vi "PNA-X control.vi"() -> ()   [LabVIEW 2020, in "VNA-Keysight PNA.lvclass"]
uses:
  VNA-Keysight PNA.lvclass
  <instrlib>/Keysight PNA Series/Keysight PNA Series.lvlib
panel:
  out "XY Graph":cluster{dbl[], dbl[]}(graph)
  in  "Sweep Points (201)":i32=201
  out "Data":dbl[](graph)
  in  "Stop Frequency (1E+10 Hz)":dbl=10000000000.0
  in  "Start Frequency (1E+6 Hz)":dbl=1000000.0
  in  "Measurement Name (MyMeas)":string="MyMeas"
  in  "Measurement Parameters (S22)":string="S22"
  in  "Channel (1)":i32=1
  in  "VISA resource name":refnum<visa-resource-name>
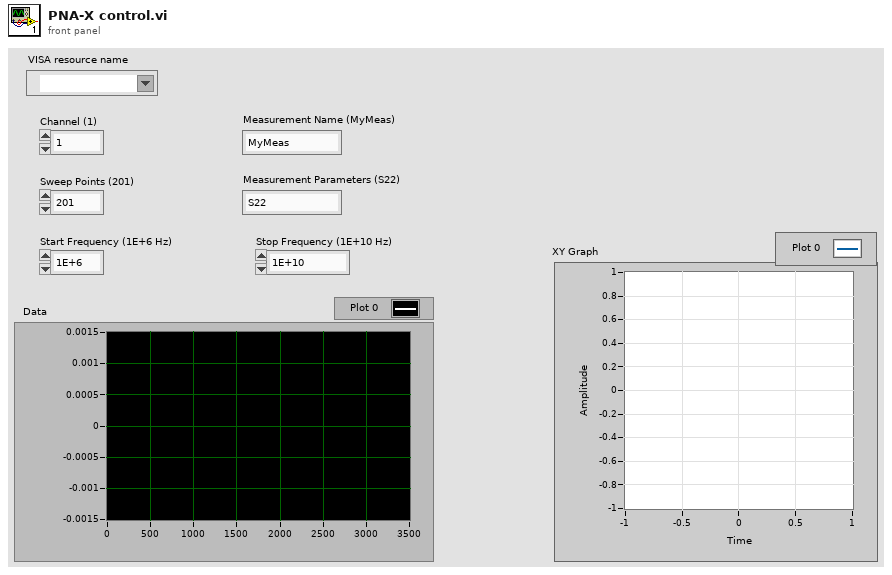
[diagram p1: front panel]
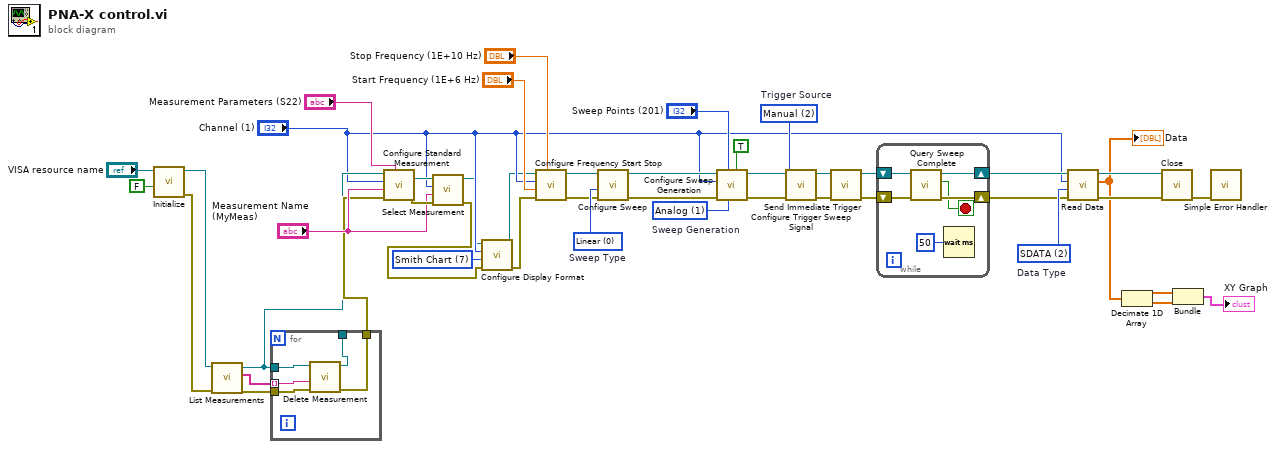
[diagram p0: block diagram]
diagram:
  w5 = 7 items=["Magnitude Linear", "Magnitude Logarithmic", "Phase", "Unwrapped phase", "Imaginary", "Real", "Polar", "Smith Chart", "Smith Admittance", "SWR", "Group Delay", "Kelvin", "Fahrenheit", "Celsius"] ("Display Format (0: Magnitude Linear)")
  w20 = 2 items=["Immediate", "External", "Manual"]  # Trigger Source
  w27 = 1 items=["Stepped", "Analog"]  # Sweep Generation
  w34 = 2 items=["FDATA", "RDATA", "SDATA", "FMEM", "SMEM", "SDIV"]  # Data Type
  w39 = 0 items=["Linear", "Logarithmic", "Power", "CW", "Segment", "Phase"]  # Sweep Type
  n1 = call <instrlib>:"Initialize.vi"("Reset (True)"=FALSE, "VISA resource name"="VISA resource name") -> ("error out"=w9:errorcluster, "VISA resource name out"=w10:refnum<visa-resource-name>)  [unwired: 8 in]
  n2 = call <instrlib>:"List Measurements.vi"("error in (no error)"=w9, "VISA resource name"=w10) -> ("error out"=w12:errorcluster, "Measurement Names"=w11:string[], "VISA resource name out"=w7:refnum<visa-resource-name>)  [unwired: 6 in, 1 out]
  n3 = for {
    tunnel: w7 -> [w50]
    tunnel: w12 -> [w49]
    tunnel: w11 -> [w48] mode=indexing
    tunnel: [w47] -> _
    tunnel: [w46] -> w8
    n4 = call <instrlib>:"Delete Measurement.vi"("error in (no error)"=w49, "Measurement Name (CH1_S11_1)"=w48, "VISA resource name"=w50) -> ("error out"=w46:errorcluster, "VISA resource name out"=w47:refnum<visa-resource-name>)  [unwired: 7 in]
  }
  n5 = call <instrlib>:"Configure Standard Measurement.vi"("Measurement Parameters (S11)"="Measurement Parameters (S22)", "error in (no error)"=w8, "Measurement Name (CH1_S11_1)"="Measurement Name (MyMeas)", "Channel (1)"="Channel (1)", "VISA resource name"=w7) -> ("error out"=w43:errorcluster, "VISA resource name out"=w42:refnum<visa-resource-name>)  [unwired: 5 in]
  n6 = call <instrlib>:"Select Measurement.vi"("error in (no error)"=w43, "Measurement Name (CH1_S11_1)"="Measurement Name (MyMeas)", "Channel (1)"="Channel (1)", "VISA resource name"=w42) -> ("error out"=w3:errorcluster, "VISA resource name out"=w4:refnum<visa-resource-name>)  [unwired: 6 in]
  n7 = call <instrlib>:"Configure Display Format.vi"("error in (no error)"=w3, "Display Format (0: Magnitude Linear)"=w5, "Channel (1)"="Channel (1)", "VISA resource name"=w4) -> ("error out"=w2:errorcluster, "VISA resource name out"=w1:refnum<visa-resource-name>)  [unwired: 6 in]
  n8 = call <instrlib>:"Configure Frequency Start Stop.vi"("Stop Frequency (2E+6 Hz)"="Stop Frequency (1E+10 Hz)", "error in (no error)"=w2, "Start Frequency (1E+6 Hz)"="Start Frequency (1E+6 Hz)", "Channel (1)"="Channel (1)", "VISA resource name"=w1) -> ("error out"=w25:errorcluster, "VISA resource name out"=w26:refnum<visa-resource-name>)  [unwired: 5 in]
  n9 = call <instrlib>:"Configure Sweep.vi"("error in (no error)"=w25, "Sweep Type (0: Linear)"=w39, "VISA resource name"=w26) -> ("error out"=w33:errorcluster, "VISA resource name out"=w32:refnum<visa-resource-name>)  [unwired: 7 in]
  n10 = call <instrlib>:"Configure Sweep Generation.vi"("Auto Sweep or Dwell Time (T: Enable)"=TRUE ("Enable Auto Sweep/Dwell Time (T: Enable)"), "Sweep Generation (1: Analog)"=w27, "Sweep Points (201)"="Sweep Points (201)", "error in (no error)"=w33, "Channel (1)"="Channel (1)", "VISA resource name"=w32) -> ("error out"=w24:errorcluster, "VISA resource name out"=w22:refnum<visa-resource-name>)  [unwired: 4 in]
  n11 = call <instrlib>:"Configure Trigger Sweep Signal.vi"("error in (no error)"=w24, "Trigger Source (0: Immediate)"=w20, "VISA resource name"=w22) -> ("error out"=w19:errorcluster, "VISA resource name out"=w18:refnum<visa-resource-name>)  [unwired: 7 in]
  n12 = call <instrlib>:"Send Immediate Trigger.vi"("error in (no error)"=w19, "VISA resource name"=w18) -> ("error out"=w23:errorcluster, "VISA resource name out"=w21:refnum<visa-resource-name>)  [unwired: 8 in]
  n13 = while {
    shift-right: [w55] -> w29
    shift-left: w23 -> [w56]
    shift-right: [w52] -> w28
    shift-left: w21 -> [w53]
    stop <- w54 stop-if-true
    n14 = call <instrlib>:"Query Sweep Complete.vi"("error in (no error)"=w56, "VISA resource name"=w53) -> ("error out"=w55:errorcluster, "Sweep Complete"=w54:bool, "VISA resource name out"=w52:refnum<visa-resource-name>)  [unwired: 7 in]
    n15 = Wait (ms)(milliseconds to wait=u32 50) -> ()  [unwired: 1 out]
  }
  n16 = call <instrlib>:"Read Data.vi"("error in (no error)"=w29, "Data Type (0: FDATA)"=w34, "Channel (1)"="Channel (1)", "VISA resource name"=w28) -> ("error out"=w36:errorcluster, "Data"=w16:dbl[], "VISA resource name out"=w35:refnum<visa-resource-name>)  [unwired: 5 in]
  "Data" <- w16
  n17 = Decimate 1D Array(w16) -> (w15:dbl[], w14:dbl[])
  n18 = call <instrlib>:"Close.vi"("error in (no error)"=w36, "VISA resource name"=w35) -> ("error out"=w44:errorcluster)  [unwired: 9 in]
  n19 = Bundle(w15, w14) -> (→"XY Graph":cluster{dbl[], dbl[]})  [unwired: 1 in]
  n20 = call <vilib>:"Simple Error Handler.vi"("error in (no error)"=w44) -> ()  [unwired: 4 in, 5 out]
